vi "main-fan-switch.vi"(7 "LabVIEW Web Service Request":refnum<class "Web Request.lvclass">, 11 "state":bool) -> ()   [LabVIEW 2023]
uses:
  Actuators.vi
  <vilib>/wsapi/Web Request.lvclass
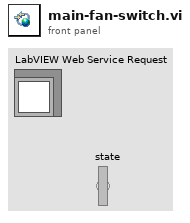
[diagram p1: front panel]
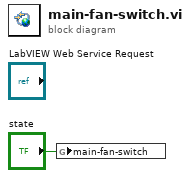
[diagram p0: block diagram]
diagram:
  n1 = global write "Actuators.vi" "main-fan-switch"("state") -> ()
